vi "Sequence Auton Parameters.vi"(8 "error in (no error)":errorcluster, 9 "Parse Parameters?":bool, 10 "Number of Parameters":i32, 11 "Auton Parameters":T1) -> (0 "error out":errorcluster, 3 "Auton Sequence":T2)   [LabVIEW 2015]
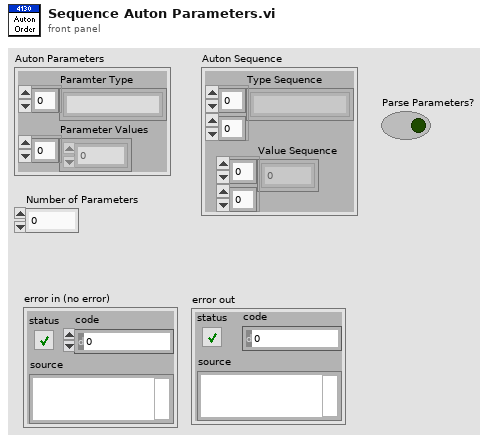
[diagram p1: front panel]
types:
  T1 = cluster{"Paramter Type":string[], "Parameter Values":dbl[]}
  T2 = cluster{"Type Sequence":string[][], "Value Sequence":dbl[][]}
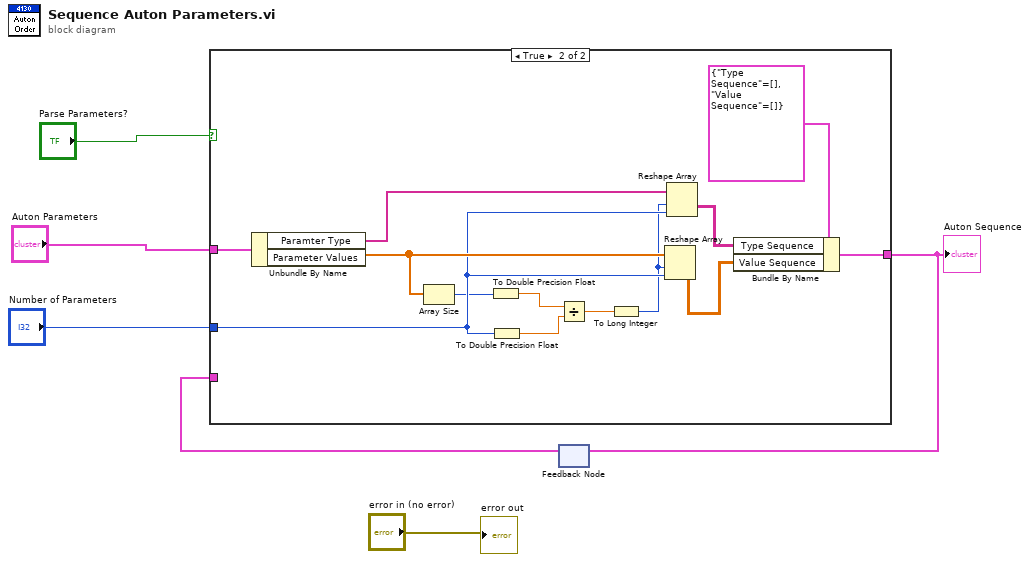
[diagram p0: block diagram]
diagram:
  n1 = feedback #1() -> (w4:T2)  [unwired: 1 in]
  n2 = case shown="True" "Parse Parameters?" {
    tunnel: "Auton Parameters" -> [_ w18]
    tunnel: [w7 w17] -> w3
    tunnel: "Number of Parameters" -> [_ w14]
    tunnel: w4 -> [w7 _]
    frame False {
    }
    frame True {
      n3 = Unbundle By Name(w18) -> ("Paramter Type"=w19:string[], "Parameter Values"=w20:dbl[])
      n4 = Array Size(array=w20) -> (size(s)=w9:i32)
      n5 = To Double Precision Float(number=w9) -> (double precision float=w11:dbl)
      n6 = To Double Precision Float(number=w14) -> (double precision float=w12:dbl)
      n7 = Divide(x=w11, y=w12) -> (x/y=w10:dbl)
      n8 = To Long Integer(number=w10) -> (32bit integer=w13:i32)
      n9 = Reshape Array(w20, w13, w14) -> (w16:dbl[][])
      n10 = Reshape Array(w19, w13, w14) -> (w15:string[][])
      n11 = Bundle By Name(cluster=T2 {"Type Sequence"=[], "Value Sequence"=[]}, "Type Sequence"=w15, "Value Sequence"=w16) -> (w17:T2)
    }
  }
  "Auton Sequence" <- w3
  n12 = feedback-in #1(w3) -> ()
  "error out" <- "error in (no error)"
